vi "Example_OE2052 Control.vi"() -> ()   [LabVIEW 2011]
uses:
  <vilib>/Utility/error.llb/DialogType.ctl
panel:
  out "B_Freq":dbl
  out "B_θ":dbl
  out "B_R":dbl
  out "B_Overload":bool
  in  "Sample count":u32
  out "Zero Data?":bool
  in  "buffer":u8
  out "Queue out":errorcluster caption="error out"
  out "Queue output":refnum<queue>
  in  "IP Address":string
  in  "Timeout":u32=100
  in  "Port":u32=10001
  out "B_PLL Lock":bool
  in  "Remote Mode":u16(ring) items=["USB"=0, "RS232"=1, "Ethernet"=3]
  out "A_Freq":dbl
  out "A_θ":dbl
  out "A_R":dbl
  out "A_PLL Lock":bool
  out "A_Overload":bool
  out "Error":string
  out "Serial Versions":string
  in  "Table":T1(tab) caption="选项卡控件"
  in  "OE2052_Configure Input Filter":T2={"Input Source"=0, "Input Impedance"=0, "Input Coupling "=0, "Sample Mode"=0, "Channel"=1, "Input Range"=0} {"Input Range" items=["1.3V", "200mV", "50mV", "10mV", "2mV", "500uV", "100uV"]; "Channel" items=["A"=1, "B"=2]; "Sample Mode" items=["HF", "LF"]; "Input Coupling" items=["AC", "DC"]; "Input Impedance" items=["50Ω", "10MΩ"]; "Input Source" items=["A", "A-B"]}
  in  "OE2052_Configure Ref Phase":T3={"Reference Source"=0, "Internal Frequency(Hz)"=1000.0, "Reference Phase"=0.0, "Reference Slope"=0, "Channel"=1, "Reference Range"=0, "Reference Input"=0} {"Reference Input" items=["REF IN1", "REF IN2"]; "Reference Range" items=["HIGH", "LOW"]; "Channel" items=["Demod 1"=1, "Demod 2"=2, "Demod 3"=3, "Demod 4"=4]; "Reference Slope" items=["SINEDC", "SINE", "TTL"]; "Reference Phase" min=-180.0 max=180.0 format="%#.2g"; "Internal Frequency(Hz)" min=1e-06 max=400000000.0 format="%#.3f"; "Reference Source" items=["External", "Internal", "Self"]}
  in  "OE2052_Configure \nGain TC":T4={"Time Constant "=20.0, "Low Pass Filter Slope "=3, "Enable Sync Filter "=0, "Channel"=1} {"Channel" items=["A"=1, "B"=2]; "Enable Sync Filter" items=["OFF", "ON"]; "Low Pass Filter Slope" items=["6 dB/oct", "12 dB/oct", "18 db/oct", "24 dB/oct", "30 dB/oct", "36 dB/oct", "42 dB/oct", "48 dB/oct"]; "Time Constant" min=1e-07 max=100.0 format="%#.3f"}
  in  "OE2052_Configure Channel Out":T5={"Channel Output"=0, "Channel Source"=0, "Offset(%)"=0.0, "Expand"=1, "AUX OUT"=1.0, "Sensitivity "=24} {"Sensitivity" items=["1 nV/fA", "2 nV/fA", "5 nV/fA", "10 nV/fA", "20 nV/fA", "50 nV/fA", "100 nV/fA", "200 nV/fA", "500 nV/fA", "1 uV/pA", "2 uV/pA", "5 uV/pA", "10 uV/pA", "20 uV/pA", "50 uV/pA", "100 uV/pA", "200 uV/pA", "500 uV/pA", "1 mV/nA", "2 mV/nA", "5 mV/nA", "10 mV/nA", "20 mV/nA", "50 mV/nA", "100 mV/nA", "200 mV/nA", "500 mV/nA", "1 V/uA"]; "AUX OUT" min=-10.0 max=10.0 format="%#.3g"; "Expand" min=1 max=10000; "Offset(%)" min=-100.0 max=100.0 format="%#_5g"; "Channel Source" items=["AUXOUT", "X1", "Y1", "R1", "θ1", "X2", "Y2", "R2", "θ2", "Frequency1", "Frequency2", "AUX-IN1", "AUX-IN2", "AUX-IN3", "AUX-IN4"]; "Channel Output" items=["CH1", "CH2", "CH3", "CH4"]}
  in  "OE2052_Configure Sine Out":T6={"SineOut Amplitude (V)"=1.0, "SineOut Offset(V) "=1.0, "SineOut Unit"=0, "SineOut Impedance"=0, "Channel"=1, "SineOut Mode"=0} {"SineOut Mode" items=["OFF", "Fixed"]; "Channel" items=["A"=1, "B"=2]; "SineOut Impedance" items=["50Ω", "HiZ"]; "SineOut Unit" items=["VPP", "VRMS"]; "SineOut Offset(V)" min=-2.5 max=2.5 format="%#.3g"; "SineOut Amplitude (V)" min=1e-06 max=1.5 format="%#.3g"}
  in  "OE2052_Configure Demodulator":T7={"Harmonic"=1, "Channel"=1, "Select Source"=0, "Mode"=0} {"Mode" items=["Harmonic"]; "Select Source" items=["SIGIN1", "SIGIN2"]; "Channel" items=["Demod 1"=1, "Demod 2"=2, "Demod 3"=3, "Demod 4"=4]; "Harmonic" min=1}
  in  "OE2052_Auto Setting":T8={"Auto Range"=FALSE, "Auto Offest"=FALSE, "Auto Phase"=FALSE, "channel"=1} {"channel" items=["A"=1, "B"=2]}
  in  "Save Button":bool
  in  "file path":path
  in  "Sample Rate(S)":dbl=0.1 min=0.001 max=100.0
  out "Status":string
  in  "Connect":bool
  in  "VISA resource name":refnum<visa-resource-name>
  in  "Baud Rate (115200)":u32=921600
  # "Tel          :   +86-020-84133345\nWebsite  :   www.ssi-instrument.com\nE-mail     :   support@si-instrument.com"
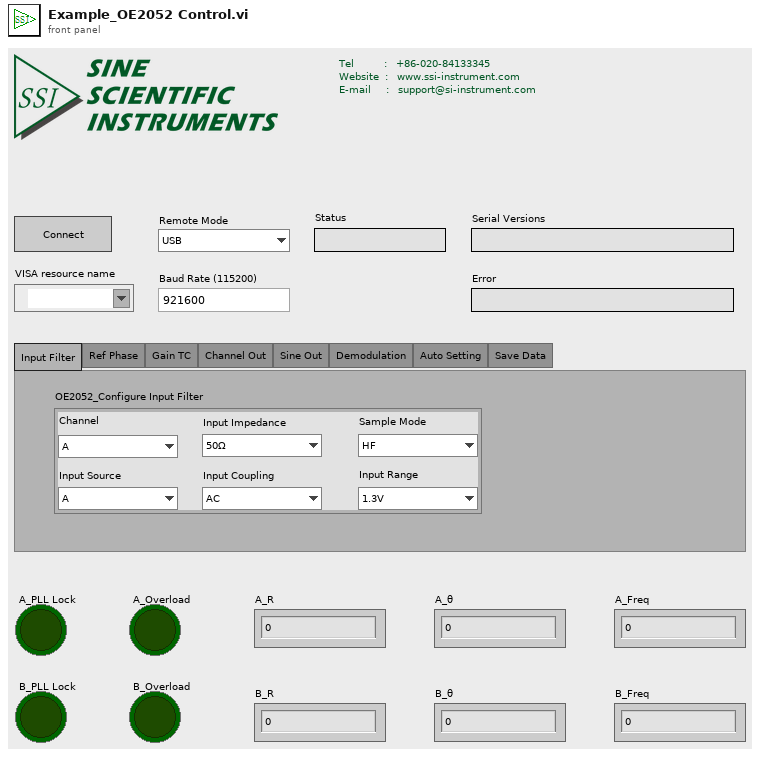
[diagram p1: front panel]
types:
  T1 = enum32{"Input Filter", "Ref Phase", "Gain TC", "Channel Out", "Sine Out", "Demodulation", "Auto Setting", "Save Data"}
  T2 = cluster{"Input Source":u16, "Input Impedance":u16, "Input Coupling ":u16, "Sample Mode":u16, "Channel":u16, "Input Range":u16}
  T3 = cluster{"Reference Source":u16, "Internal Frequency(Hz)":dbl, "Reference Phase":dbl, "Reference Slope":u16, "Channel":u16, "Reference Range":u16, "Reference Input":u16}
  T4 = cluster{"Time Constant ":dbl, "Low Pass Filter Slope ":u8, "Enable Sync Filter ":u16, "Channel":u16}
  T5 = cluster{"Channel Output":u16, "Channel Source":u16, "Offset(%)":dbl, "Expand":u16, "AUX OUT":dbl, "Sensitivity ":u16}
  T6 = cluster{"SineOut Amplitude (V)":dbl, "SineOut Offset(V) ":dbl, "SineOut Unit":u8, "SineOut Impedance":u8, "Channel":u16, "SineOut Mode":u8}
  T7 = cluster{"Harmonic":u16, "Channel":u16, "Select Source":u16, "Mode":u16}
  T8 = cluster{"Auto Range":bool, "Auto Offest":bool, "Auto Phase":bool, "channel":u16}
  T9 = enum16{"OE1022", "OE1022D", "OE1201", "OE2031&OE2041", "OE1311&OE1351", "OE2052"}
  T10 = cluster{"Port":u32, "Timeout":u32, "IP Address":string}
  T11 = cluster{"A_PLL Lock":bool, "A_Overload":bool, "B_PLL Lock":bool, "B_Overload":bool}
  T12 = cluster{"Demod 1_X":dbl, "Demod 1_Y":dbl, "Demod 1_R":dbl, "Demod 1_θ":dbl, "Demod 1_Freq":dbl, "Demod 2_X":dbl, "Demod 2_Y":dbl, "Demod 2_R":dbl, "Demod 2_θ":dbl, "Demod 2_Freq":dbl, "Demod 3_X":dbl, "Demod 3_Y":dbl, "Demod 3_R":dbl, "Demod 3_θ":dbl, "Demod 3_Freq":dbl, "Demod 4_X":dbl, "Demod 4_Y":dbl, "Demod 4_R":dbl, "Demod 4_θ":dbl, "Demod 4_Freq":dbl, "Aux_In1":dbl, "Aux_In2":dbl, "Aux_In3":dbl, "Aux_In4":dbl}
  T13 = typedef "DialogType.ctl" = u16
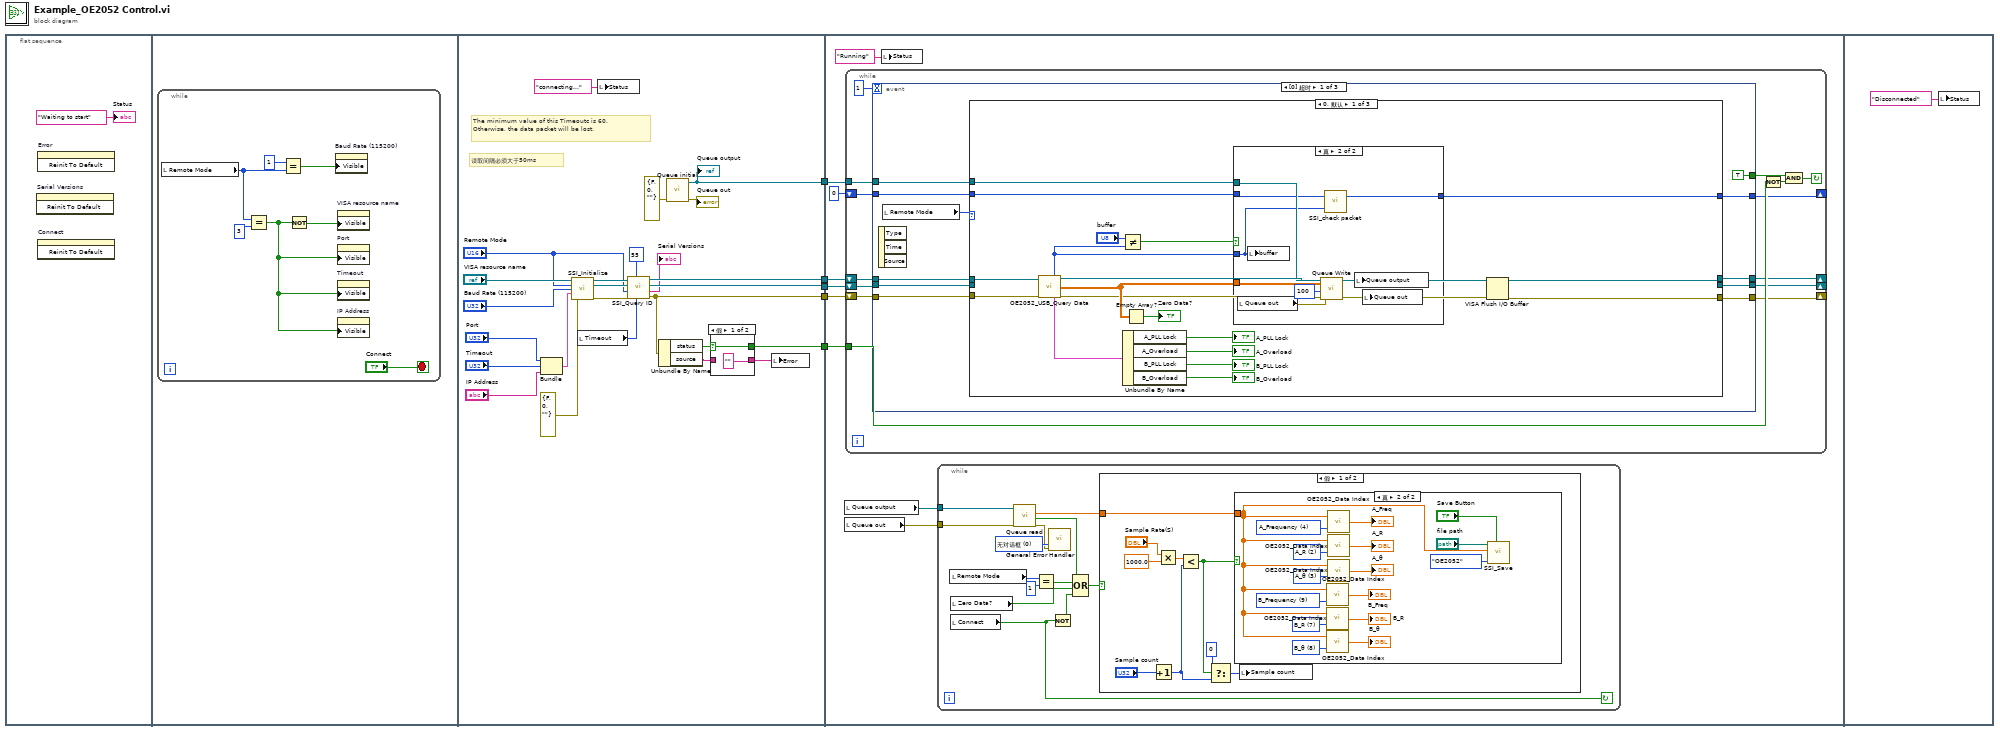
[diagram p0: block diagram]
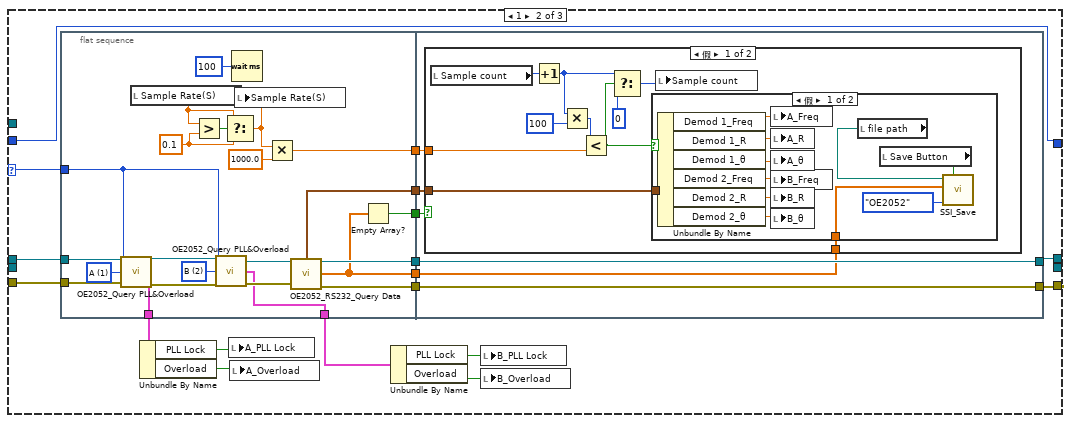
[diagram p6: hidden frame]
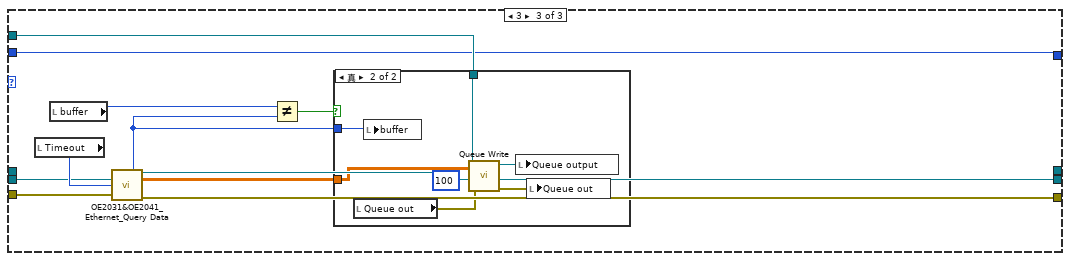
[diagram p9: hidden frame]
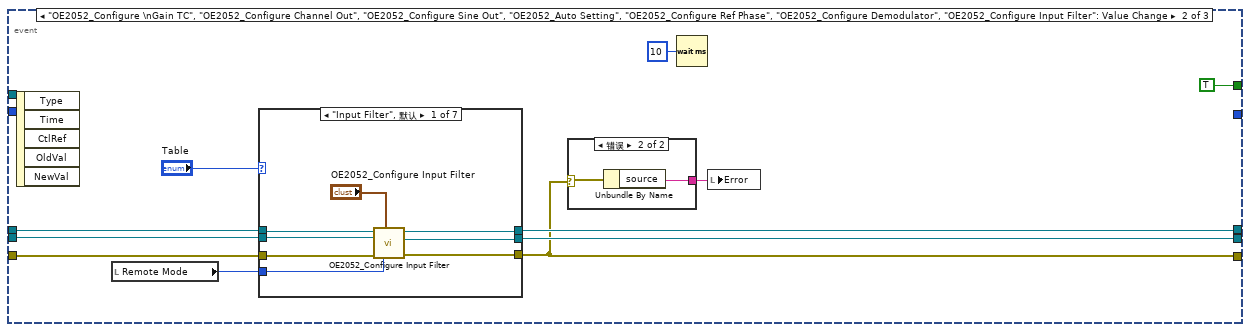
[diagram p11: hidden frame]
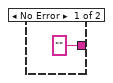
[diagram p12: hidden frame]
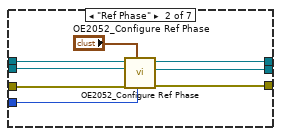
[diagram p13: hidden frame]
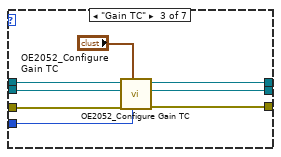
[diagram p14: hidden frame]
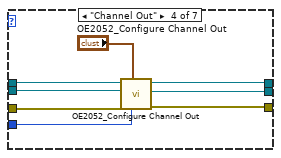
[diagram p15: hidden frame]
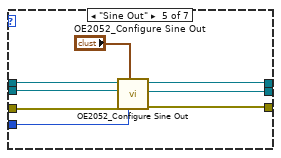
[diagram p16: hidden frame]
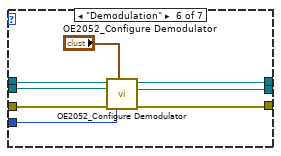
[diagram p17: hidden frame]
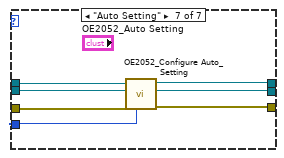
[diagram p18: hidden frame]
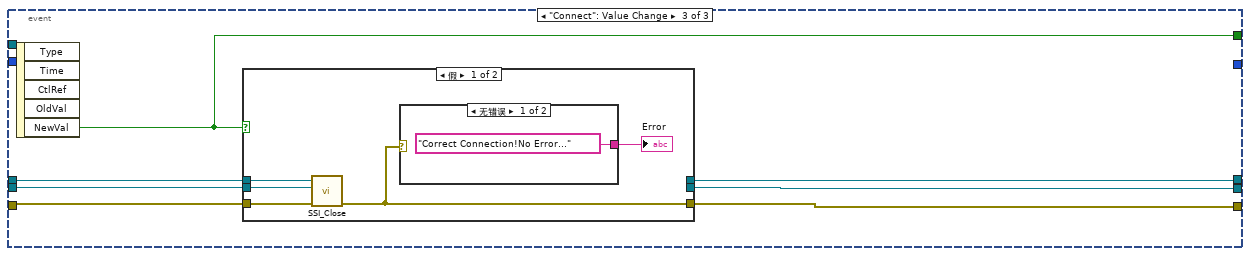
[diagram p19: hidden frame]
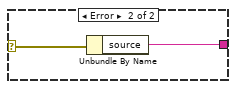
[diagram p20: hidden frame]
diagram:
  n1 = flat-sequence {
    tunnel: [w32] -> w5
    tunnel: [w31] -> w4
    tunnel: [w28] -> w3
    tunnel: [w25] -> w2
    tunnel: [w16] -> w1
    tunnel: w5 -> [w50]
    tunnel: w4 -> [w49]
    tunnel: w3 -> [w48]
    tunnel: w2 -> [w47]
    tunnel: w1 -> [w44]
    frame #0 {
      n2 = invoke on="Serial Versions" class="Str" method="Reinit To Default"() -> ()  [unwired: 3 in, 3 out]
      n3 = invoke on="Error" class="Str" method="Reinit To Default"() -> ()  [unwired: 3 in, 3 out]
      n4 = invoke on="Connect" class="Bool (严格)" method="Reinit To Default"() -> ()  [unwired: 3 in, 3 out]
      "Status" <- "Waiting to start" ("status")
    }
    frame #1 {
      n5 = while {
        stop <- "Connect" stop-if-true
        n6 = local read "Remote Mode"() -> (w8:u16)
        n7 = Equal?(x=w8, y=u16 3) -> (x = y?=w10:bool)
        n8 = Equal?(x=u16 1, y=w8) -> (x = y?=w7:bool)
        n9 = Not(x=w10) -> (.not. x?=w11:bool)
        n10 = property on="Baud Rate (115200)" class="DigNum (严格)"("Visible"=w7) -> ()  [unwired: 2 in, 2 out]
        n11 = property on="VISA resource name" class="VISAName"("Visible"=w11) -> ()  [unwired: 2 in, 2 out]
        n12 = property on="Port" class="DigNum (严格)"("Visible"=w10) -> ()  [unwired: 2 in, 2 out]
        n13 = property on="Timeout" class="DigNum (严格)"("Visible"=w10) -> ()  [unwired: 2 in, 2 out]
        n14 = property on="IP Address" class="Str"("Visible"=w10) -> ()  [unwired: 2 in, 2 out]
      }
    }
    frame #2 {
      # "读取间隔必须大于50ms"
      # "The minimum value of this Timeoutc is 60. \nOtherwise, the data packet will be lost."
      n15 = Bundle("Port"="Port", "Timeout"="Timeout", "IP Address"="IP Address") -> (w20:T10)  [unwired: 1 in]
      n16 = call "SSI_Initialize.vi"("VISA resource name"="VISA resource name", "Remote Mode"="Remote Mode", "baud rate (921600)"="Baud Rate (115200)", "Ethernet"=w20, "error in (no error)"=errorcluster {"status"=FALSE, "code"=0, "source"=""}) -> ("VISA resource name out"=w36:refnum<visa-resource-name>, "connection ID(Ethernet)"=w35:refnum<k5>, "error out"=w34:errorcluster)  [unwired: 8 in]
      n17 = local read "Timeout"() -> (w19:u32)
      n18 = local write "Status"("connecting..." ("status")) -> ()
      n19 = call "SSI_Query ID.vi"("Timeout"=w19, "Number of bytes"=u32 55, "Error in (no error)"=w34, "Remote Mode"="Remote Mode", "Connection ID in"=w35, "VISA resource name"=w36) -> ("Error out"=w28:errorcluster, "Read Buffer"=→"Serial Versions":string, "Connection ID out"=w31:refnum<k5>, "VISA resource  out"=w32:refnum<visa-resource-name>)  [unwired: 2 in]
      n20 = Unbundle By Name(w28) -> ("status"=w27:bool, "source"=w26:string)
      n21 = call "Queue initial.vi"("Error in (no error)"=errorcluster {"status"=FALSE, "code"=0, "source"=""}) -> ("Error out"=→"Queue out":errorcluster, "Queue output"=w16:refnum<queue>)  [unwired: 9 in]
      "Queue output" <- w16
      n22 = case shown="假" w27 {
        selector: w27 -> [w40 w42]
        tunnel: [w40 w42] -> w25
        tunnel: ["" w41] -> w24
        tunnel: w26 -> [_ w41]
        frame False {
        }
        frame True {
        }
      }
      n23 = local write "Error"(w24) -> ()
    }
    frame #3 {
      n24 = local read "Queue output"() -> (w46:refnum<queue>)
      n25 = local read "Queue out"() -> (w45:errorcluster)
      n26 = while {
        tunnel: w47 -> [w99]
        tunnel: w44 -> [w95]
        shift-right: [w92] -> _
        shift-left: w48 -> [w96]
        shift-right: [w93] -> _
        shift-left: w49 -> [w97]
        shift-right: [w94] -> _
        shift-left: w50 -> [w98]
        shift-right: [w90] -> _
        shift-left: 0 -> [w91]
        stop <- w100 continue-if-true
        n27 = event shown="[0] 超时" {
          selector: _ -> [_ _ _]
          dyn-events: _ -> [_ _ _]
          timeout: 1 -> [_ _ _]
          tunnel: [TRUE ("Stop") TRUE ("Stop") w299] -> w101
          tunnel: [w114 w231 w302] -> w92
          tunnel: [w113 w236 w301] -> w94
          tunnel: [w112 w235 w300] -> w93
          tunnel: w98 -> [w108 w239 w305]
          tunnel: w97 -> [w106 w238 w304]
          tunnel: w96 -> [w107 w237 w303]
          tunnel: w95 -> [w109 _ _]
          tunnel: w91 -> [w105 _ _]
          tunnel: [w104 _ _] -> w90
          event Timeout {
            n28 = event-data() -> ()  [unwired: 1 in, 3 out]
            n29 = local read "Remote Mode"() -> (w110:u16)
            n30 = case shown="0, 默认" w110 {
              selector: w110 -> [_ w157 _]
              tunnel: [w122 w159 w220] -> w114
              tunnel: [w125 w158 _] -> w113
              tunnel: [_ _ w221] -> w112
              tunnel: w109 -> [w133 _ w219]
              tunnel: w108 -> [w124 w161 _]
              tunnel: w107 -> [w123 w160 w213]
              tunnel: w106 -> [_ _ w214]
              tunnel: w105 -> [w116 w144 w212]
              tunnel: [w115 w144 w212] -> w104
              frame 0, Default {
                n31 = call "OE2052_USB_Query Data.vi"("VISA resource name"=w124, "Error in (no error)"=w123) -> ("Buffer Count"=w130:u8, "VISA resource  out"=w127:refnum<visa-resource-name>, "Total Data Array"=w129:dbl[][], "A&B_PLL&Overload"=w117:T11, "Error out"=w126:errorcluster)  [unwired: 7 in, 2 out]
                n32 = Not Equal?(x="buffer", y=w130) -> (x != y?=w131:bool)
                n33 = Unbundle By Name(w117) -> ("A_PLL Lock"=→"A_PLL Lock":bool, "A_Overload"=→"A_Overload":bool, "B_PLL Lock"=→"B_PLL Lock":bool, "B_Overload"=→"B_Overload":bool)
                n34 = Empty Array?(array=w129) -> (empty?=→"Zero Data?":bool)
                n35 = case shown="真" w131 {
                  tunnel: w129 -> [_ w138]
                  tunnel: w133 -> [_ w142]
                  tunnel: w130 -> [_ w135]
                  tunnel: w116 -> [w134 w137]
                  tunnel: [w134 w136] -> w115
                  frame False {
                  }
                  frame True {
                    n36 = local read "Queue out"() -> (w139:errorcluster)
                    n37 = local write "buffer"(w135) -> ()
                    n38 = call "Queue Write.vi"("Error in (no error)"=w139, "Group Count"=100, "Input Array"=w138, "Queue Input"=w142) -> ("Error out"=w140:errorcluster, "Queue output"=w141:refnum<queue>)  [unwired: 6 in]
                    n39 = call "SSI_check packet.vi"("input"=w135, "input loss"=w137) -> ("loss count"=w136:i32)  [unwired: 1 out]
                    n40 = local write "Queue output"(w141) -> ()
                    n41 = local write "Queue out"(w140) -> ()
                  }
                }
                n42 = VISA Flush I/O Buffer(VISA resource name=w127, error in (no error)=w126) -> (VISA resource name out=w125:refnum<visa-resource-name>, error out=w122:errorcluster)  [unwired: 1 in]
              }
              frame 1 {
                n43 = flat-sequence {
                  tunnel: [w176] -> w156
                  tunnel: [w177] -> w155
                  tunnel: [w180] -> w154
                  tunnel: [w179] -> w153
                  tunnel: [w175] -> w152
                  tunnel: [w171] -> w151
                  tunnel: w161 -> [w170]
                  tunnel: w160 -> [w169]
                  tunnel: w157 -> [w164]
                  tunnel: [w163] -> w150
                  tunnel: [w162] -> w147
                  tunnel: w156 -> [w189]
                  tunnel: w155 -> [w190]
                  tunnel: [w190] -> w158
                  tunnel: [w189] -> w159
                  tunnel: w154 -> [w186]
                  tunnel: w153 -> [w185]
                  tunnel: w152 -> [w187]
                  tunnel: w151 -> [w188]
                  frame #0 {
                    w165 = u16 2 items=["A"=1, "B"=2] ("channel")
                    w166 = u16 1 items=["A"=1, "B"=2] ("channel")
                    w183 = 0.1 ("y")
                    n44 = call "OE2052_Query PLL&Overload.vi"("VISA resource name"=w170, "channel"=w166, "Remote Mode"=w164, "Error in (no error)"=w169) -> ("VISA resource  out"=w167:refnum<visa-resource-name>, "OE2052_Query \nPLL&Overload"=w163:cluster{"PLL Lock":bool, "Overload":bool}, "Error out"=w168:errorcluster)  [unwired: 7 in, 2 out]
                    n45 = local read "Sample Rate(S)"() -> (w178:dbl)
                    n46 = Greater?(x=w178, y=w183) -> (0:w182:bool)
                    n47 = call "OE2052_Query PLL&Overload.vi"("VISA resource name"=w167, "channel"=w165, "Remote Mode"=w164, "Error in (no error)"=w168) -> ("VISA resource  out"=w174:refnum<visa-resource-name>, "OE2052_Query \nPLL&Overload"=w162:cluster{"PLL Lock":bool, "Overload":bool}, "Error out"=w173:errorcluster)  [unwired: 7 in, 2 out]
                    n48 = Select(t=w178, s=w182, f=w183) -> (s? t:f=w181:dbl)
                    n49 = Wait (ms)(milliseconds to wait=u32 100 ("等待时间（毫秒）")) -> ()  [unwired: 1 out]
                    n50 = local write "Sample Rate(S)"(w181) -> ()
                    n51 = Multiply(x=w181, y=1000.0) -> (x*y=w179:dbl)
                    n52 = call "OE2052_RS232_Query Data.vi"("VISA resource name"=w174, "Error in (no error)"=w173) -> ("VISA resource  out"=w177:refnum<visa-resource-name>, "Data Array"=w171:dbl[], "Parameter Values"=w175:T12, "Error out"=w176:errorcluster)  [unwired: 9 in, 1 out]
                    n53 = Empty Array?(array=w171) -> (empty?=w180:bool)
                  }
                  frame #1 {
                    n54 = case shown="假" w186 {
                      tunnel: w188 -> [w200 _]
                      tunnel: w187 -> [w199 _]
                      tunnel: w185 -> [w195 _]
                      frame False {
                        n55 = local read "Sample count"() -> (w198:u32)
                        n56 = Increment(x=w198) -> (x+1=w194:u32)
                        n57 = Multiply(x=w194, y=u32 100) -> (x*y=w196:u32)
                        n58 = Less?(x=w196, y=w195) -> (x < y?=w193:bool)
                        n59 = Select(t=w194, s=w193, f=0) -> (s? t:f=w192:u32)
                        n60 = case shown="假" w193 {
                          tunnel: w199 -> [w211 _]
                          tunnel: w200 -> [w207 _]
                          frame False {
                            n61 = Unbundle By Name(w211) -> ("Demod 1_Freq"=w210:dbl, "Demod 1_R"=w209:dbl, "Demod 1_θ"=w208:dbl, "Demod 2_Freq"=w203:dbl, "Demod 2_R"=w201:dbl, "Demod 2_θ"=w202:dbl)
                            n62 = local write "A_Freq"(w210) -> ()
                            n63 = local write "A_R"(w209) -> ()
                            n64 = local write "A_θ"(w208) -> ()
                            n65 = local write "B_Freq"(w203) -> ()
                            n66 = local write "B_R"(w201) -> ()
                            n67 = local write "B_θ"(w202) -> ()
                            n68 = local read "file path"() -> (w206:path)
                            n69 = local read "Save Button"() -> (w205:bool)
                            n70 = call "SSI_Save.vi"("file path (dialog if empty)"=w206, "1D data"=w207, "Instrument Mode"=T9."OE2052", "Save Button"=w205) -> ()  [unwired: 7 in]
                          }
                          frame True {
                          }
                        }
                        n71 = local write "Sample count"(w192) -> ()
                      }
                      frame True {
                      }
                    }
                  }
                }
                n72 = Unbundle By Name(w150) -> ("PLL Lock"=w148:bool, "Overload"=w149:bool)
                n73 = local write "A_PLL Lock"(w148) -> ()
                n74 = local write "A_Overload"(w149) -> ()
                n75 = Unbundle By Name(w147) -> ("PLL Lock"=w146:bool, "Overload"=w145:bool)
                n76 = local write "B_PLL Lock"(w146) -> ()
                n77 = local write "B_Overload"(w145) -> ()
              }
              frame 3 {
                n78 = local read "Timeout"() -> (w222:u32)
                n79 = local read "buffer"() -> (w217:u8)
                n80 = call "OE2031&OE2041_Ethernet_Query Data.vi"("Connection ID in"=w214, "Timeout"=w222, "Error in (no error)"=w213) -> ("Buffer Count"=w216:u8, "Connection ID out"=w221:refnum<k5>, "Total Data Array"=w215:dbl[][], "Error out"=w220:errorcluster)  [unwired: 5 in, 4 out]
                n81 = Not Equal?(x=w217, y=w216) -> (x != y?=w218:bool)
                n82 = case shown="真" w218 {
                  tunnel: w219 -> [_ w228]
                  tunnel: w216 -> [_ w224]
                  tunnel: w215 -> [_ w223]
                  frame False {
                  }
                  frame True {
                    n83 = local read "Queue out"() -> (w225:errorcluster)
                    n84 = local write "buffer"(w224) -> ()
                    n85 = call "Queue Write.vi"("Error in (no error)"=w225, "Group Count"=100, "Input Array"=w223, "Queue Input"=w228) -> ("Error out"=w226:errorcluster, "Queue output"=w227:refnum<queue>)  [unwired: 6 in]
                    n86 = local write "Queue output"(w227) -> ()
                    n87 = local write "Queue out"(w226) -> ()
                  }
                }
              }
            }
          }
          event "OE2052_Configure \nGain TC", "OE2052_Configure Channel Out", "OE2052_Configure Sine Out", "OE2052_Auto Setting", "OE2052_Configure Ref Phase", "OE2052_Configure Demodulator", "OE2052_Configure Input Filter": Value Change {
            n88 = event-data() -> ()  [unwired: 1 in, 5 out]
            n89 = local read "Remote Mode"() -> (w234:u16)
            n90 = case shown="\"Input Filter\", 默认" "Table" {
              tunnel: w239 -> [w250 w259 w267 w272 w279 w288 w298]
              tunnel: w238 -> [w249 w258 w265 w273 w278 w289 w297]
              tunnel: w237 -> [w251 w257 w266 w275 w283 w291 w296]
              tunnel: [w246 w256 w263 w269 w280 w287 w294] -> w236
              tunnel: [w247 w255 w264 w271 w282 w286 w292] -> w231
              tunnel: [w248 w254 w262 w270 w281 w285 w293] -> w235
              tunnel: w234 -> [w245 w253 w261 w274 w277 w290 w295]
              frame "Input Filter", Default {
                n91 = call "OE2052_Configure Input Filter.vi"("OE2052_Configure Input Filter"="OE2052_Configure Input Filter", "Error in (no error)"=w251, "Remote Mode"=w245, "Connection ID in"=w249, "VISA resource name"=w250) -> ("Error out"=w247:errorcluster, "Connection ID out"=w248:refnum<k5>, "VISA resource  out"=w246:refnum<visa-resource-name>)  [unwired: 3 in, 1 out]
              }
              frame "Ref Phase" {
                n92 = call "OE2052_Configure Ref Phase.vi"("OE2052_Configure Ref Phase"="OE2052_Configure Ref Phase", "Error in (no error)"=w257, "Remote Mode"=w253, "Connection ID in"=w258, "VISA resource name"=w259) -> ("Error out"=w255:errorcluster, "Connection ID out"=w254:refnum<k5>, "VISA resource  out"=w256:refnum<visa-resource-name>)  [unwired: 3 in, 1 out]
              }
              frame "Gain TC" {
                n93 = call "OE2052_Configure Gain TC.vi"("OE2052_Configure \nGain TC"="OE2052_Configure \nGain TC", "Error in (no error)"=w266, "Remote Mode"=w261, "Connection ID in"=w265, "VISA resource name"=w267) -> ("Error out"=w264:errorcluster, "Connection ID out"=w262:refnum<k5>, "VISA resource  out"=w263:refnum<visa-resource-name>)  [unwired: 3 in, 1 out]
              }
              frame "Channel Out" {
                n94 = call "OE2052_Configure Channel Out.vi"("OE2052_Configure Channel Out"="OE2052_Configure Channel Out", "Error in (no error)"=w275, "Remote Mode"=w274, "Connection ID in"=w273, "VISA resource name"=w272) -> ("Error out"=w271:errorcluster, "Connection ID out"=w270:refnum<k5>, "VISA resource  out"=w269:refnum<visa-resource-name>)  [unwired: 3 in, 1 out]
              }
              frame "Sine Out" {
                n95 = call "OE2052_Configure Sine Out.vi"("OE2052_Configure Sine Out"="OE2052_Configure Sine Out", "Error in (no error)"=w283, "Remote Mode"=w277, "Connection ID in"=w278, "VISA resource name"=w279) -> ("Error out"=w282:errorcluster, "Connection ID out"=w281:refnum<k5>, "VISA resource  out"=w280:refnum<visa-resource-name>)  [unwired: 3 in, 1 out]
              }
              frame "Demodulation" {
                n96 = call "OE2052_Configure Demodulator.vi"("OE2052_Configure Demodulator"="OE2052_Configure Demodulator", "Error in (no error)"=w291, "Remote Mode"=w290, "Connection ID in"=w289, "VISA resource name"=w288) -> ("Error out"=w286:errorcluster, "Connection ID out"=w285:refnum<k5>, "VISA resource  out"=w287:refnum<visa-resource-name>)  [unwired: 3 in, 1 out]
              }
              frame "Auto Setting" {
                n97 = call "OE2052_Configure Auto_Setting.vi"("Error in (no error)"=w296, "Remote Mode"=w295, "Connection ID in"=w297, "VISA resource name"=w298) -> ("Error out"=w292:errorcluster, "Connection ID out"=w293:refnum<k5>, "VISA resource  out"=w294:refnum<visa-resource-name>)  [unwired: 4 in, 1 out]
              }
            }
            n98 = case shown="错误" w231 {
              selector: w231 -> [_ w243]
              tunnel: ["" ("source") w242] -> w232
              frame No Error {
              }
              frame Error {
                n99 = Unbundle By Name(w243) -> ("source"=w242:string)
              }
            }
            n100 = Wait (ms)(milliseconds to wait=u32 10 ("等待时间（毫秒）")) -> ()  [unwired: 1 out]
            n101 = local write "Error"(w232) -> ()
          }
          event "Connect": Value Change {
            n102 = event-data() -> ("NewVal"=w299:bool)  [unwired: 1 in, 4 out]
            n103 = case shown="假" w299 {
              tunnel: w305 -> [w310 w315]
              tunnel: w304 -> [w309 w314]
              tunnel: w303 -> [w308 w316]
              tunnel: [w307 w316] -> w302
              tunnel: [_ w315] -> w301
              tunnel: [_ w314] -> w300
              frame False {
                n104 = call "SSI_Close.vi"("Error in (no error)"=w308, "Connection ID in"=w309, "VISA resource name"=w310) -> ("Error out"=w307:errorcluster)  [unwired: 4 in]
                n105 = case shown="无错误" w307 {
                  selector: w307 -> [_ w313]
                  tunnel: ["Correct Connection!No Error..." ("source") w312] -> w306
                  frame No Error {
                  }
                  frame Error {
                    n106 = Unbundle By Name(w313) -> ("source"=w312:string)
                  }
                }
                "Error" <- w306
              }
              frame True {
              }
            }
          }
        }
        n107 = Not(x=w99) -> (.not. x?=w102:bool)
        n108 = And(x=w101, y=w102) -> (x .and. y?=w100:bool)
      }
      n109 = local write "Status"("Running" ("status")) -> ()
      n110 = while {
        tunnel: w46 -> [w57]
        tunnel: w45 -> [w56]
        stop <- w52 continue-if-true
        w59 = T13 0 items=["无对话框", "确定信息", "继续或停止信息", "确定信息＋警告", "继续/停止+警告"] ("type of dialog (OK msg:1)")
        n111 = local read "Remote Mode"() -> (w64:u16)
        n112 = local read "Zero Data?"() -> (w60:bool)
        n113 = local read "Connect"() -> (w52:bool)
        n114 = call "Queue read.vi"("Error in (no error)"=w56, "Queue Input"=w57) -> ("Error out"=w58:errorcluster, "Timeout？"=w54:bool, "Output Array"=w55:sgl[])  [unwired: 7 in]
        n115 = Equal?(x=w64, y=u16 1) -> (x = y?=w61:bool)
        n116 = call <vilib>:"General Error Handler.vi"("type of dialog (OK msg:1)"=w59, "error in (no error)"=w58) -> ()  [unwired: 9 in, 5 out]
        n117 = Not(x=w52) -> (.not. x?=w53:bool)
        n118 = Compound Arithmetic op=OR(w54, w61, w60, w53) -> (w62:bool)
        n119 = case shown="假" w62 {
          tunnel: w55 -> [w73 _]
          frame False {
            n120 = Increment(x="Sample count") -> (x+1=w67:u32)
            n121 = Multiply(x="Sample Rate(S)", y=1000.0) -> (x*y=w71:dbl)
            n122 = Less?(x=w71, y=w67) -> (x < y?=w68:bool)
            n123 = Select(t=0, s=w68, f=w67) -> (s? t:f=w66:u32)
            n124 = case shown="真" w68 {
              tunnel: w73 -> [_ w77]
              frame False {
              }
              frame True {
                w78 = u16 8 items=["A_X", "A_Y", "A_R", "A_θ", "A_Frequency", "B_X", "B_Y", "B_R", "B_θ", "B_Frequency"] ("Parameter Type")
                w79 = u16 7 items=["A_X", "A_Y", "A_R", "A_θ", "A_Frequency", "B_X", "B_Y", "B_R", "B_θ", "B_Frequency"] ("Parameter Type")
                w80 = u16 9 items=["A_X", "A_Y", "A_R", "A_θ", "A_Frequency", "B_X", "B_Y", "B_R", "B_θ", "B_Frequency"] ("Parameter Type")
                w81 = u16 3 items=["A_X", "A_Y", "A_R", "A_θ", "A_Frequency", "B_X", "B_Y", "B_R", "B_θ", "B_Frequency"] ("Parameter Type")
                w82 = u16 2 items=["A_X", "A_Y", "A_R", "A_θ", "A_Frequency", "B_X", "B_Y", "B_R", "B_θ", "B_Frequency"] ("Parameter Type")
                w83 = u16 4 items=["A_X", "A_Y", "A_R", "A_θ", "A_Frequency", "B_X", "B_Y", "B_R", "B_θ", "B_Frequency"] ("Parameter Type")
                n125 = call "OE2052_Data Index.vi"("Parameter Type"=w80, "Input Date Array"=w77) -> ("Parameter"=→"B_Freq":dbl)
                n126 = call "OE2052_Data Index.vi"("Parameter Type"=w79, "Input Date Array"=w77) -> ("Parameter"=→"B_R":dbl)
                n127 = call "OE2052_Data Index.vi"("Parameter Type"=w78, "Input Date Array"=w77) -> ("Parameter"=→"B_θ":dbl)
                n128 = call "OE2052_Data Index.vi"("Parameter Type"=w83, "Input Date Array"=w77) -> ("Parameter"=→"A_Freq":dbl)
                n129 = call "OE2052_Data Index.vi"("Parameter Type"=w82, "Input Date Array"=w77) -> ("Parameter"=→"A_R":dbl)
                n130 = call "OE2052_Data Index.vi"("Parameter Type"=w81, "Input Date Array"=w77) -> ("Parameter"=→"A_θ":dbl)
                n131 = call "SSI_Save.vi"("file path (dialog if empty)"="file path", "1D data"=w77, "Instrument Mode"=T9."OE2052", "Save Button"="Save Button") -> ()  [unwired: 7 in]
              }
            }
            n132 = local write "Sample count"(w66) -> ()
          }
          frame True {
          }
        }
      }
    }
    frame #4 {
      n133 = local write "Status"("Disconnected" ("status")) -> ()
    }
  }
